vi "QR.vi"(8 "error in (no error)":errorcluster, 10 "Image":T2, 11 "client handle":T1) -> (1 "value":cluster{"id":string, "hora_entrada":string}, 2 "client handle out":T1, 3 "QR Imagen":T2(plugin-control))   [LabVIEW 2025]
uses:
  <vilib>/httpClient/ClientHandle.ctl
  <vilib>/vision/Image Controls.llb/IMAQ Image.ctl
  <vilib>/httpClient/LabVIEWHTTPClient.lvlib
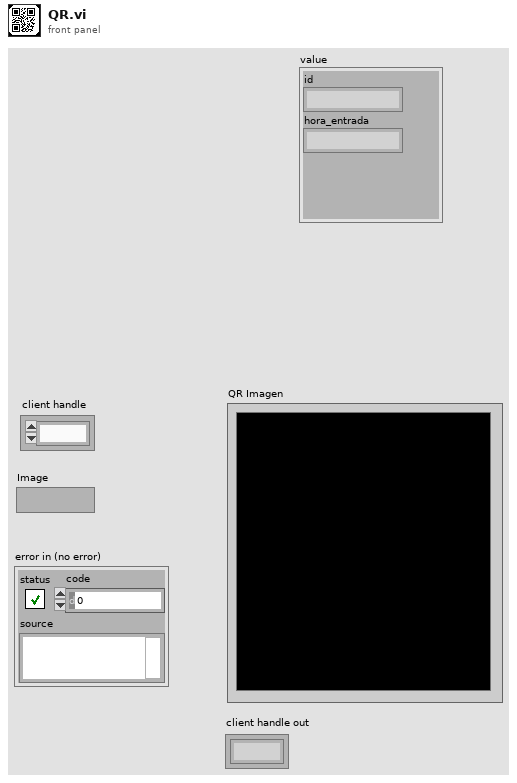
[diagram p1: front panel]
types:
  T1 = typedef "LabVIEWHTTPClient.lvlib/ClientHandle.ctl" = refnum<k1>
  T2 = typedef "IMAQ Image.ctl" = refnum<image>
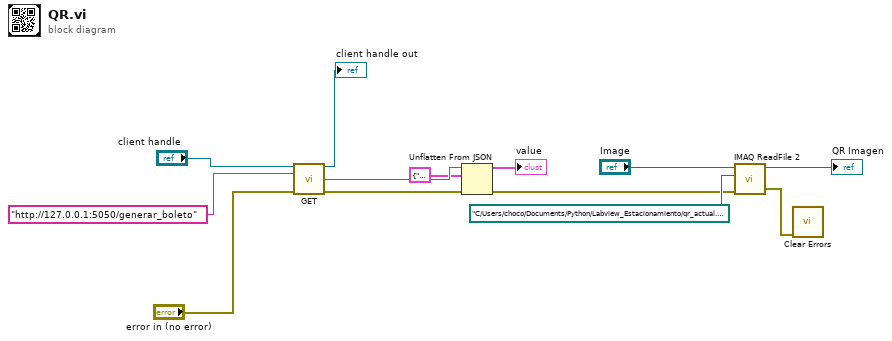
[diagram p0: block diagram]
diagram:
  n1 = call <vilib>:"GET.vi"("client handle"="client handle", "url"="http://127.0.0.1:5050/generar_boleto", "error in (no error)"="error in (no error)") -> ("client handle out"=→"client handle out":T1, "body"=w3:string, "error out"=w5:errorcluster)  [unwired: 9 in, 1 out]
  n2 = Unflatten From JSON(JSON string=w3, type and defaults=cluster{"hora_entrada":string, "id":string} {"hora_entrada"="", "id"=""}, error in (no error)=w5) -> (value=→"value":cluster{"hora_entrada":string, "id":string}, error out=w4:errorcluster)  [unwired: 4 in]
  n3 = call "IMAQ ReadFile 2"("File Path"=path "C:/Users/choco/Documents/Python/Labview_Estacionamiento/qr_actual.png", "error in (no error)"=w4, "Image"="Image") -> ("error out"=w13:errorcluster, "Image Out"=→"QR Imagen":T2)  [unwired: 4 in, 3 out]
  n4 = call <vilib>:"Clear Errors.vi"("error in (no error)"=w13) -> ()  [unwired: 5 in, 2 out]
